vi "Set Channel Default Value.vi"(8 "error in (no error)":errorcluster, 9 "Dimensions":T1={"Row"=1, "Column"=1}, 10 "Default Value":dbl[][](array[numeric])=[[0.0]], 11 "Channel Reference in":u64 format="%.0x") -> (0 "error out":errorcluster, 3 "Channel Reference out":u64 format="%.0x")   [LabVIEW 2013, in "Hierarchy Framework.lvlib" / "Channel.lvclass"]
doc: "Sets the <B>Default Value</B> for the channel specified by <B>Channel Reference in</B>. The channel retains the <B>Default Value</B> until it receives a new value.The Dimension default value is {1,1},that means it is a single point channel."
uses:
  Channel.lvclass
  Ctls/Dimensions.ctl
  Generic/Generic.lvclass
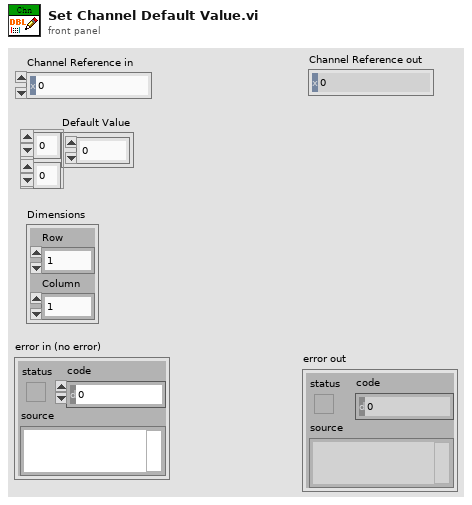
[diagram p1: front panel]
types:
  T1 = typedef "Hierarchy Framework.lvlib/Channel.lvclass/Dimensions.ctl" = cluster{"Row":i32, "Column":i32}
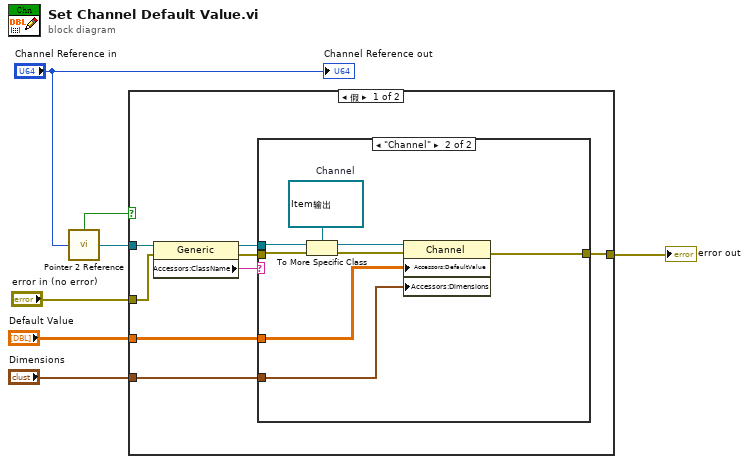
[diagram p0: block diagram]
diagram:
  n1 = call "Pointer 2 Reference.vi"("Pointer"="Channel Reference in") -> ("Not A Refnum?"=w6:bool, "Generic Reference"=w5:refnum<data-value>)
  n2 = case shown="假" w6 {
    tunnel: w5 -> [w15 _]
    tunnel: "error in (no error)" -> [w12 w25]
    tunnel: [w10 w25] -> w3
    tunnel: "Default Value" -> [w9 _]
    tunnel: "Dimensions" -> [w8 _]
    frame False {
      n3 = property class="Generic"(reference=w15, error in=w12) -> (reference out=w13:refnum<data-value>, error out=w11:errorcluster, "Accessors:ClassName"=w14:string)
      n4 = case shown="\"Channel\"" w14 {
        tunnel: w13 -> [_ w24]
        tunnel: w11 -> [w16 w23]
        tunnel: [w16 w19] -> w10
        tunnel: w9 -> [_ w18]
        tunnel: w8 -> [_ w17]
        frame Default {
        }
        frame "Channel" {
          w22 = refnum<data-value> refnum  # Channel
          n5 = To More Specific Class(target class=w22, reference=w24, error in=w23) -> (specific class reference=w21:refnum<data-value>, error out=w20:errorcluster)
          n6 = property class="Channel"(reference=w21, error in=w20, "Accessors:DefaultValue"=w18, "Accessors:Dimensions"=w17) -> (error out=w19:errorcluster)  [unwired: 1 out]
        }
      }
    }
    frame True {
    }
  }
  "error out" <- w3
  "Channel Reference out" <- "Channel Reference in"
